vi "BoxToSetting.vi"(9 "GridSize":dbl=5.0, 10 "Line":dbl[](array[numeric])=[30.0, 30.0, 50.0, 50.0, 15.0], 11 "Scan Settings":T1={"XStart"=-150000000, "XEnd"=150000000, "XNum"=350, "YStart"=-150000000, "YEnd"=150000000, "YNum"=500, "ZStart"=-30000, "ZEnd"=30000, "ZNum"=30}) -> (3 "Settings":i32[][](array[numeric]))   [LabVIEW 2014]
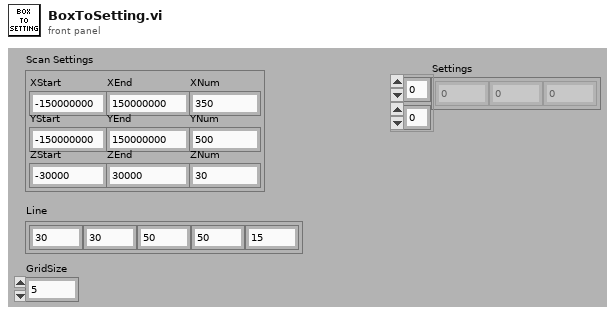
[diagram p1: front panel]
types:
  T1 = cluster{"XStart":i32, "XEnd":i32, "XNum":i32, "YStart":i32, "YEnd":i32, "YNum":i32, "ZStart":i32, "ZEnd":i32, "ZNum":i32}
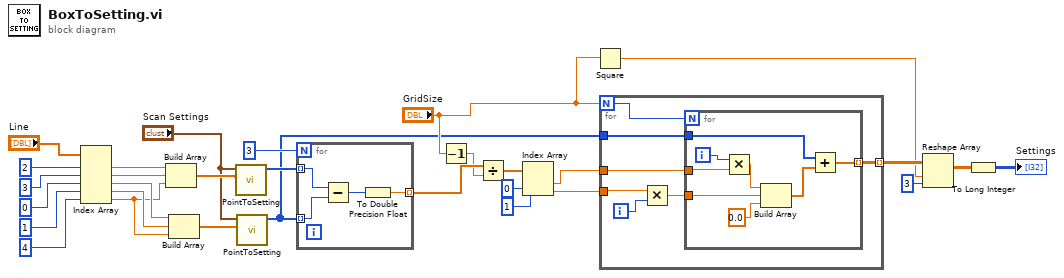
[diagram p0: block diagram]
diagram:
  n1 = Index Array(array="Line", index #1=2 ("index"), index #2=3 ("index"), index #3=0 ("index"), index #4=1 ("index"), index #5=4 ("index")) -> (element #1=w24:dbl, element #2=w23:dbl, element #3=w22:dbl, element #4=w21:dbl, element #5=w20:dbl)
  n2 = Build Array(w24, w23, w20) -> (w9:dbl[])
  n3 = Build Array(w22, w21, w20) -> (w7:dbl[])
  n4 = call "PointToSetting.vi"("Clicked"=w9, "Scan Settings"="Scan Settings") -> ("Setting"=w10:i32[])  [unwired: 9 in]
  n5 = call "PointToSetting.vi"("Clicked"=w7, "Scan Settings"="Scan Settings") -> ("Setting"=w6:i32[])  [unwired: 9 in]
  n6 = for {
    N: 3 -> [_]
    tunnel: w10 -> [w34] mode=indexing
    tunnel: w6 -> [w33] mode=indexing
    tunnel: [w31] -> w18 mode=indexing
    n7 = Subtract(x=w34, y=w33) -> (x-y=w32:i32)
    n8 = To Double Precision Float(number=w32) -> (double precision float=w31:dbl)
  }
  n9 = Decrement(x="GridSize") -> (x-1=w11:dbl)
  n10 = Divide(x=w18, y=w11) -> (x/y=w5:dbl[])
  n11 = Index Array(array=w5, index #1=0 ("index"), index #2=1 ("index")) -> (element #1=w2:dbl, element #2=w1:dbl)
  n12 = Square(x="GridSize") -> (x^2=w15:dbl)
  n13 = for {
    N: "GridSize" -> [w39]
    tunnel: w6 -> [w41]
    tunnel: w2 -> [w38]
    tunnel: [w40] -> w17 mode=indexing
    tunnel: w1 -> [w37]
    i -> [w36]
    n14 = Multiply(x=w37, y=w36) -> (x*y=w35:dbl)
    n15 = for {
      N: w39 -> [_]
      tunnel: w41 -> [w44]
      tunnel: w38 -> [w49]
      tunnel: [w43] -> w40 mode=indexing
      tunnel: w35 -> [w45]
      i -> [w48]
      n16 = Multiply(x=w48, y=w49) -> (x*y=w46:dbl)
      n17 = Build Array(w46, w45, 0.0 ("element")) -> (w42:dbl[])
      n18 = Add(x=w44, y=w42) -> (x+y=w43:dbl[])
    }
  }
  n19 = Reshape Array(w17, w15, 3 ("dimension size")) -> (w14:dbl[][])
  n20 = To Long Integer(number=w14) -> (32bit integer=→"Settings":i32[][])
